vi "Temperature Monitor.vi"() -> ()   [LabVIEW 2010]
panel:
  out "Waveform Graph":dbl[](graph)
  in  "While Loop Delay":dbl(knob) scale=0.0..2.0
  in  "stop":bool
  out "String":string
  in  "Unit":bool
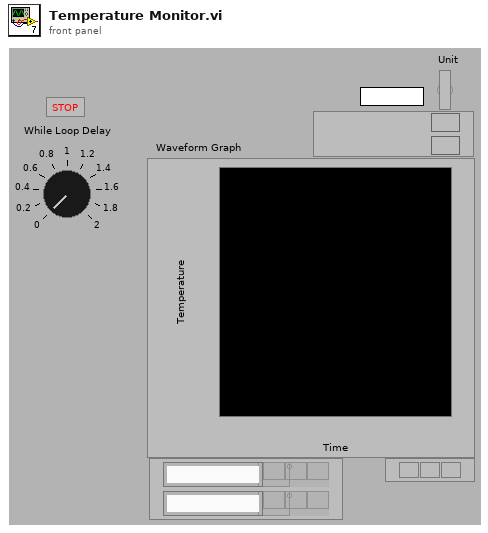
[diagram p1: front panel]
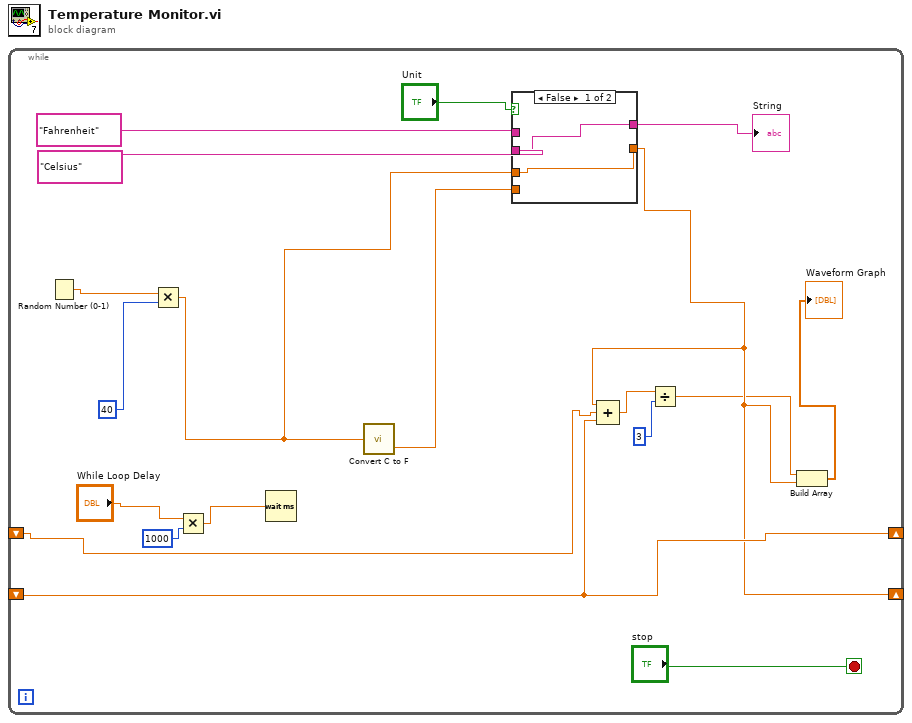
[diagram p0: block diagram]
diagram:
  n1 = while {
    shift-right: [w4] -> _
    shift-left: _ -> [w5]
    shift-right: [w3] -> _
    shift-left: _ -> [w4]
    stop <- "stop" stop-if-true
    n2 = Random Number (0-1)() -> (number: 0 to 1=w19:dbl)
    n3 = Multiply(x=w19, y=40) -> (x*y=w17:dbl)
    n4 = Multiply(x="While Loop Delay", y=1000) -> (x*y=w8:dbl)
    n5 = Wait (ms)(milliseconds to wait=w8) -> ()  [unwired: 1 out]
    n6 = call "Convert C to F.vi"("Temp in C"=w17) -> ("Temp in F"=w16:dbl)  [unwired: 1 in]
    n7 = case shown="False" "Unit" {
      tunnel: w17 -> [w21 _]
      tunnel: w16 -> [_ w23]
      tunnel: [w21 w23] -> w3
      tunnel: "Celsius" -> [w20 _]
      tunnel: "Fahrenheit" -> [_ w22]
      tunnel: [w20 w22] -> w12
      frame False {
      }
      frame True {
      }
    }
    "String" <- w12
    n8 = Compound Arithmetic op=ADD(w3, w5, w4) -> (w6:dbl)
    n9 = Divide(x=w6, y=3) -> (x/y=w2:dbl)
    n10 = Build Array(w2, w3) -> (→"Waveform Graph":dbl[])
  }
